vi "DAQmx Reset Device.vi"(0 "device in":tag, 11 "error in":errorcluster) -> (15 "error out":errorcluster)   [LabVIEW 2011]
doc: "Immediately aborts all active tasks associated with a device, disconnects any routes, and returns the device to an initialized state. Aborting a task immediately terminates the currently active operation, such as a read or a write. Aborting a task puts the task into an unstable but recoverable state. To recover the task, use DAQmx Start to restart the task or use DAQmx Stop to reset the task without starting it."
uses:
  nilvaiu.dll
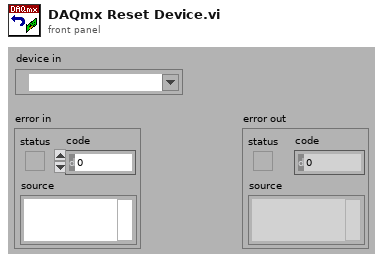
[diagram p1: front panel]
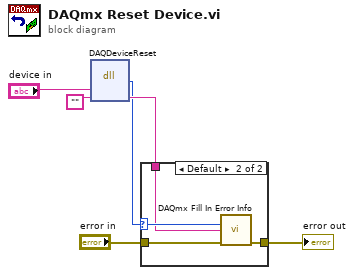
[diagram p0: block diagram]
diagram:
  n1 = dll-call lib="nilvaiu.dll" fn="DAQDeviceReset"("deviceID"="device in", "extendedErrorInfo"="") -> (w1:i32, "extendedErrorInfo"=w2:string)  [unwired: 4 in, 2 out]
  n2 = case shown="Default" w1 {
    selector: w1 -> [_ w9]
    tunnel: "error in" -> [w7 w11]
    tunnel: [w7 w10] -> w5
    tunnel: w2 -> [_ w8]
    frame 0 {
    }
    frame Default {
      n3 = call "DAQmx Fill In Error Info.vi"("status code"=w9, "extended error info"=w8, "error in"=w11) -> ("error out"=w10:errorcluster)  [unwired: 1 in, 11 out]
    }
  }
  "error out" <- w5
